vi "MetaClient.vi"(8 "error in (no error)":errorcluster) -> (0 "error out":errorcluster, 3 "params_from_server":cluster{"steps":i32, "runs":i32}, 4 "Stop?":bool=TRUE)   [LabVIEW 2017]
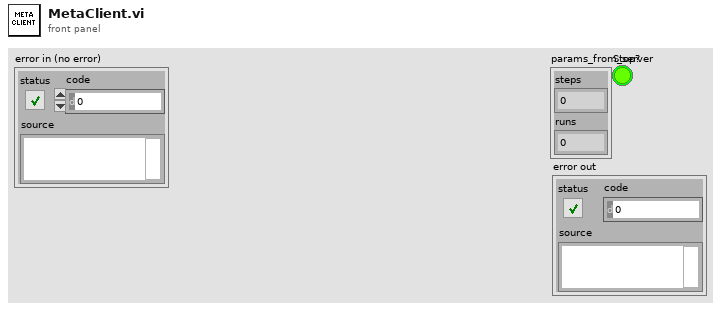
[diagram p1: front panel]
types:
  T1 = enum16{"Standard", "Buffered", "CRLF", "Immediate"}
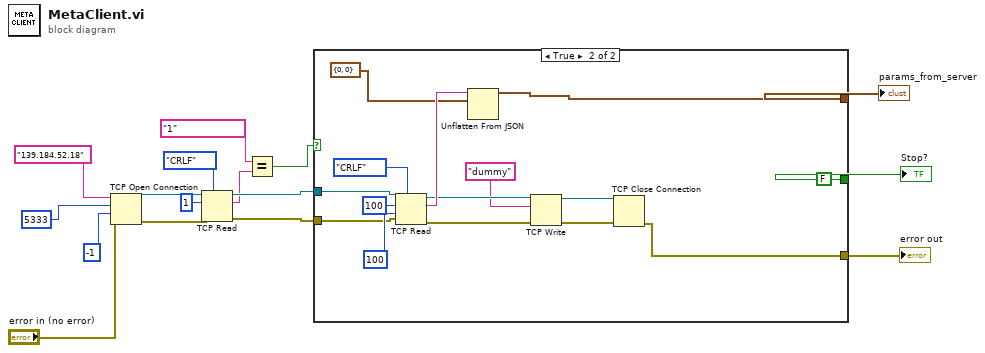
[diagram p0: block diagram]
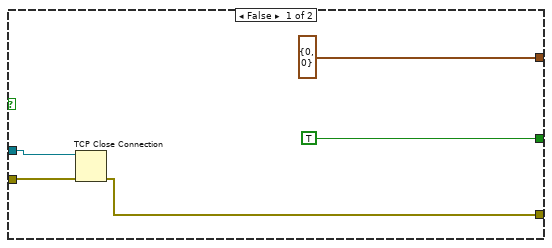
[diagram p2: hidden frame]
diagram:
  n1 = TCP Open Connection(address="139.184.52.18", remote port or service name=u16 5333, timeout ms (60000)=-1, error in (no error)="error in (no error)") -> (connection ID=w6:refnum<k5>, error out=w5:errorcluster)  [unwired: 1 in]
  n2 = TCP Read(connection ID=w6, bytes to read=1, error in (no error)=w5, 7:T1."CRLF" ("mode (standard)")) -> (connection ID out=w12:refnum<k5>, data out=w10:string, error out=w11:errorcluster)  [unwired: 1 in]
  n3 = Equal?(x="1", y=w10) -> (x = y?=w8:bool)
  n4 = case shown="True" w8 {
    tunnel: w12 -> [w20 w31]
    tunnel: w11 -> [w21 w30]
    tunnel: [cluster{"steps":i32, "runs":i32} {"steps"=0, "runs"=0} w29] -> w7
    tunnel: [TRUE FALSE] -> w3
    tunnel: [w17 w22] -> w1
    frame False {
      n5 = TCP Close Connection(connection ID=w20, error in (no error)=w21) -> (error out=w17:errorcluster)  [unwired: 1 in, 1 out]
    }
    frame True {
      n6 = TCP Read(connection ID=w31, bytes to read=100, error in (no error)=w30, 7:T1."CRLF" ("mode (standard)"), 9:100 ("timeout ms (25000)")) -> (connection ID out=w27:refnum<k5>, data out=w35:string, error out=w26:errorcluster)
      n7 = Unflatten From JSON(JSON string=w35, type and defaults=cluster{"steps":i32, "runs":i32} {"steps"=0, "runs"=0}) -> (value=w29:cluster{"steps":i32, "runs":i32})  [unwired: 5 in, 1 out]
      n8 = TCP Write(connection ID=w27, data in="dummy", error in (no error)=w26) -> (connection ID out=w23:refnum<k5>, error out=w24:errorcluster)  [unwired: 1 in, 1 out]
      n9 = TCP Close Connection(connection ID=w23, error in (no error)=w24) -> (error out=w22:errorcluster)  [unwired: 1 in, 1 out]
    }
  }
  "params_from_server" <- w7
  "Stop?" <- w3
  "error out" <- w1
